vi "measure_current_keithley-2450.vi"(7 "error in (no error)":errorcluster, 10 "VISA resource name":refnum<visa-resource-name>="GPIB1::24::INSTR") -> (0 "error out":errorcluster, 2 "Data":string[](array[string]))   [LabVIEW 2016]
uses:
  <instrlib>/Keithley 2450/Keithley 2450.lvlib
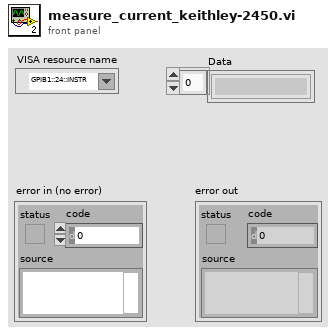
[diagram p1: front panel]
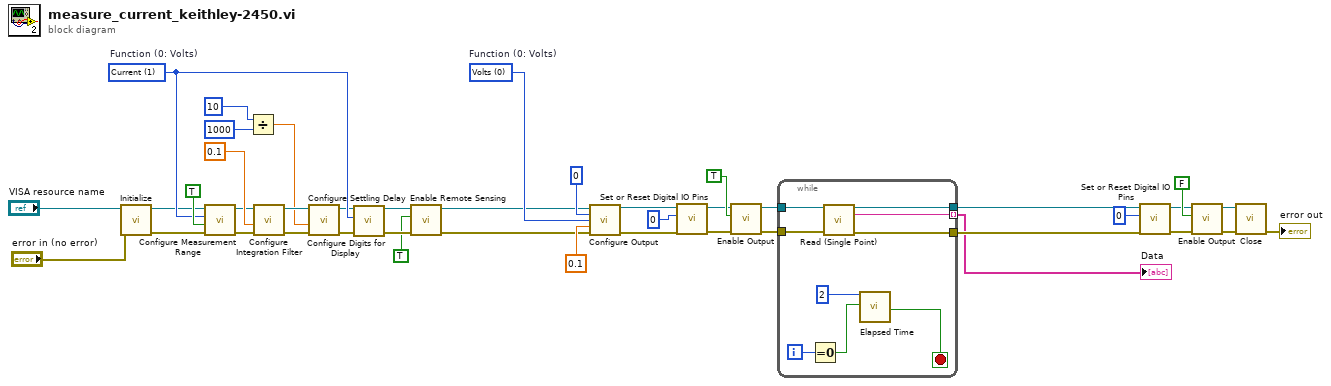
[diagram p0: block diagram]
diagram:
  w13 = u16 0 items=["Volts", "Current", "Resistance"]  # Function (0: Volts)
  w37 = u16 1 items=["Volts", "Current", "Resistance"]  # Function (0: Volts)
  n1 = call <instrlib>:"Initialize.vi"("error in (no error)"="error in (no error)", "VISA resource name"="VISA resource name") -> ("error out"=w27:errorcluster, "VISA resource name out"=w28:refnum<visa-resource-name>)  [unwired: 8 in]
  n2 = call <instrlib>:"Configure Measurement Range.vi"("error in (no error)"=w27, "Enable Auto Range (T:Enable)"=TRUE, "Function (0: Volts)"=w37, "VISA resource name"=w28) -> ("error out"=w30:errorcluster, "VISA resource name out"=w29:refnum<visa-resource-name>)  [unwired: 6 in]
  n3 = Divide(x=10, y=1000) -> (x/y=w36:dbl)
  n4 = call <instrlib>:"Configure Integration Filter.vi"("error in (no error)"=w30, "Measurement Speed (1 PLC)"=0.1, "VISA resource name"=w29) -> ("error out"=w39:errorcluster, "VISA resource name out"=w38:refnum<visa-resource-name>)  [unwired: 7 in]
  n5 = call <instrlib>:"Configure Settling Delay.vi"("error in (no error)"=w39, "Manual Delay (0 sec)"=w36, "VISA resource name"=w38) -> ("error out"=w34:errorcluster, "VISA resource name out"=w33:refnum<visa-resource-name>)  [unwired: 7 in]
  n6 = call <instrlib>:"Configure Digits for Display.vi"("error in (no error)"=w34, "Function (0: Volts)"=w37, "VISA resource name"=w33) -> ("error out"=w32:errorcluster, "VISA resource name out"=w31:refnum<visa-resource-name>)  [unwired: 7 in]
  n7 = call <instrlib>:"Enable Remote Sensing.vi"("error in (no error)"=w32, "Enable Remote Sensing (T: Enable)"=TRUE, "VISA resource name"=w31) -> ("error out"=w2:errorcluster, "VISA resource name out"=w3:refnum<visa-resource-name>)  [unwired: 7 in]
  n8 = call <instrlib>:"Configure Output.vi"("VISA resource name"=w3, "Source Level (0)"=0, "Source Mode  (0: Voltage)"=w13, "Source Limit Level (0.1)"=0.1 ("Compliance  Level"), "error in (no error)"=w2) -> ("VISA resource name out"=w9:refnum<visa-resource-name>, "error out"=w8:errorcluster)  [unwired: 9 in]
  n9 = call <instrlib>:"Set or Reset Digital IO Pins.vi"("error in (no error)"=w8, "Digital IO Line (1)"=0 ("Numeric"), "VISA resource name"=w9) -> ("error out"=w6:errorcluster, "VISA resource name out"=w7:refnum<visa-resource-name>)  [unwired: 7 in]
  n10 = call <instrlib>:"Enable Output.vi"("error in (no error)"=w6, "Enable Output (T: Enable)"=TRUE ("Output (Off)"), "VISA resource name"=w7) -> ("error out"=w23:errorcluster, "VISA resource name out"=w24:refnum<visa-resource-name>)  [unwired: 7 in]
  n11 = while {
    tunnel: w24 -> [w51]
    tunnel: w23 -> [w50]
    tunnel: [w49] -> w18
    tunnel: [w44] -> w15
    tunnel: [w43] -> w1 mode=indexing
    i -> [w47]
    stop <- w48 stop-if-true
    n12 = Equal To 0?(x=w47) -> (x = 0?=w46:bool)
    n13 = call <instrlib>:"Read (Single Point).vi"("VISA resource name"=w51, "error in (no error)"=w50) -> ("VISA resource name out"=w49:refnum<visa-resource-name>, "Data out"=w43:string, "error out"=w44:errorcluster)  [unwired: 11 in]
    n14 = call "Elapsed Time"("Time Target (s)"=2, "Reset"=w46) -> ("Time has Elapsed"=w48:bool)  [unwired: 10 in, 7 out]
  }
  "Data" <- w1
  n15 = call <instrlib>:"Set or Reset Digital IO Pins.vi"("error in (no error)"=w15, "Digital IO Line (1)"=0, "VISA resource name"=w18) -> ("error out"=w14:errorcluster, "VISA resource name out"=w19:refnum<visa-resource-name>)  [unwired: 7 in]
  n16 = call <instrlib>:"Enable Output.vi"("error in (no error)"=w14, "Enable Output (T: Enable)"=FALSE ("Output (Off)"), "VISA resource name"=w19) -> ("error out"=w21:errorcluster, "VISA resource name out"=w22:refnum<visa-resource-name>)  [unwired: 7 in]
  n17 = call <instrlib>:"Close.vi"("error in (no error)"=w21, "VISA resource name"=w22) -> ("error out"=→"error out":errorcluster)  [unwired: 9 in]
